vi "CC System Message.vi"(8 "error in (no error)":errorcluster, 11 "Message":string) -> (0 "error out":errorcluster)   [LabVIEW 2021]
uses:
  Subsystems/SS cluster Data Queue type.ctl
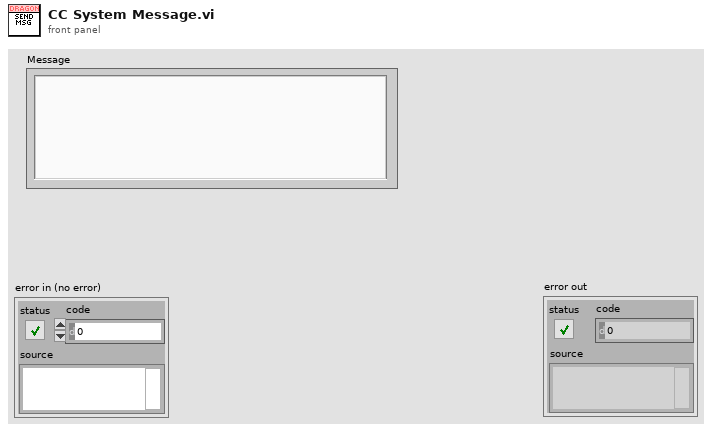
[diagram p1: front panel]
types:
  T1 = typedef "SS cluster Data Queue type.ctl" = cluster{"Source":string, "Type":string, "Data":variant}
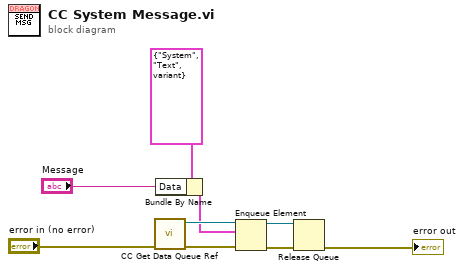
[diagram p0: block diagram]
diagram:
  n1 = call "CC Get Data Queue Ref.vi"("error in (no error)"="error in (no error)") -> ("error out"=w5:errorcluster, "Data Q"=w6:refnum<queue>)  [unwired: 9 in]
  n2 = Bundle By Name(cluster=T1 {"Source"="System", "Type"="Text", "Data"=variant} ("element"), "Data"="Message") -> (w2:T1)
  n3 = Enqueue Element(queue=w6, element=w2, error in (no error)=w5) -> (queue out=w9:refnum<queue>, error out=w8:errorcluster)  [unwired: 1 in, 1 out]
  n4 = Release Queue(queue=w9, error in (no error)=w8) -> (error out=→"error out":errorcluster)  [unwired: 1 in, 2 out]
